vi "Frequency_Counter_TTi_SoftFP.vi"(0 "reference in":refnum<class "Frequency_Counter_TTi.lvclass">, 2 "Floating":bool, 5 "error in (no error)":errorcluster) -> (14 "reference out":refnum<class "Frequency_Counter_TTi.lvclass">, 19 "error out":errorcluster)   [LabVIEW 2022 SP3, in "Frequency_Counter_TTi.lvlib" / "Frequency_Counter_TTi.lvclass"]
uses:
  Frequency_Counter_TTi.lvclass
  <vilib>/numeric/Random Number (Range) DBL.vi
  Components/ViPER.lvlibp/ViPER.lvclass
  <vilib>/measure/NI_MABase.lvlib
  C:/Projects/Medulla/ViPER/Examples/Flux_Capacitor_Tester/Components/ViPER.lvlibp/ViPER.lvclass
panel:
  in  "Measure":bool
  out "Waveform Graph":waveform(dbl)(graph)
  out "Freq MHz":dbl format="%.4f"
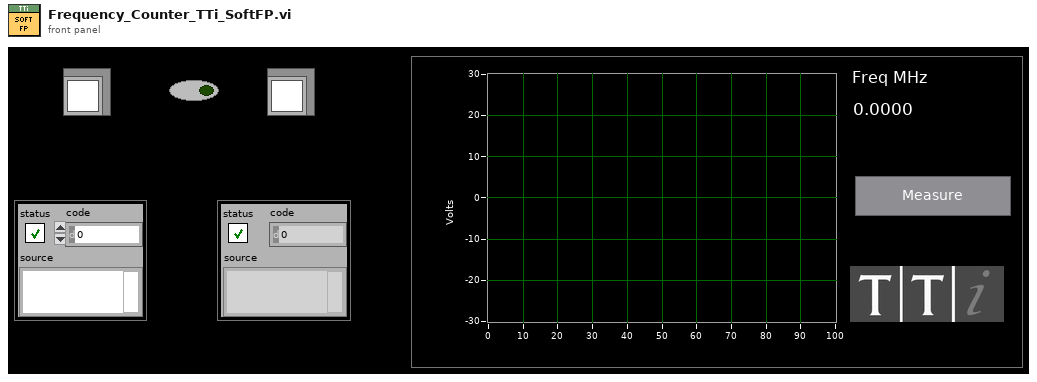
[diagram p1: front panel]
types:
  T1 = enum32{"Invalid", "Standard", "Closed", "Hidden", "Minimized", "Maximized"}
  T2 = enum16{"Sine Wave", "Triangle Wave", "Square Wave", "Sawtooth Wave"}[]
  T3 = typedef "Frequency_Counter_TTi.lvlib/Frequency_Counter_TTi.lvclass/ObjectAttributes.ctl" = cluster{"Config":T4, "Freq":dbl}
  T4 = typedef "Frequency_Counter_TTi.lvlib/Frequency_Counter_TTi.lvclass/Config.ctl" = cluster{"ComPort":refnum<visa-resource-name>}
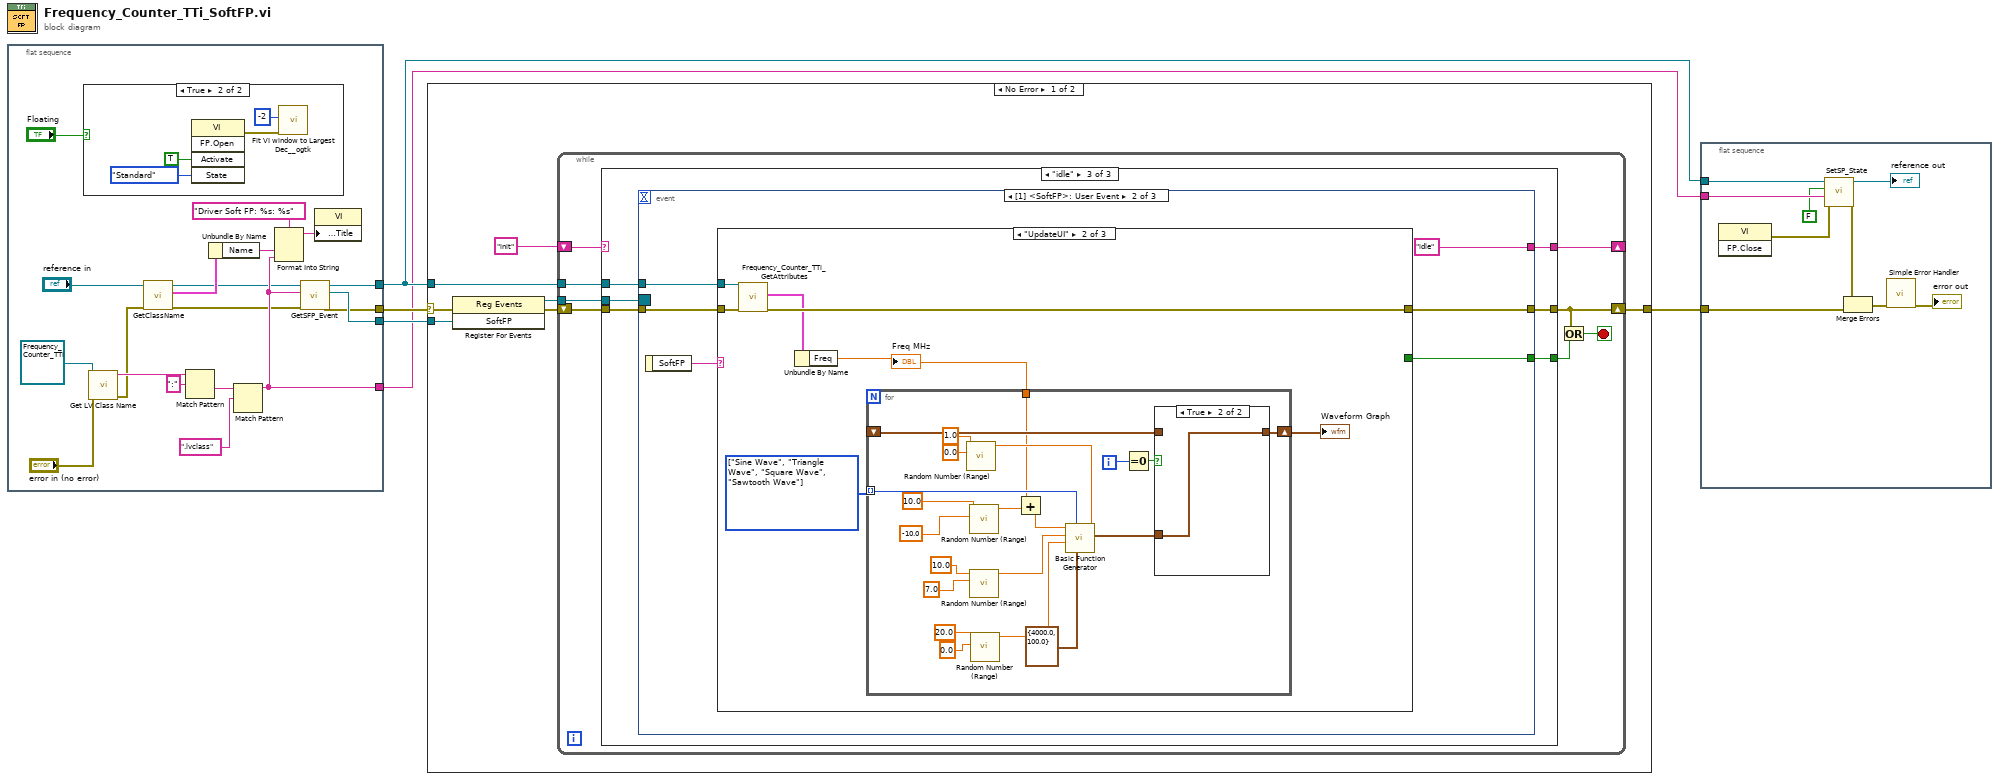
[diagram p0: block diagram]
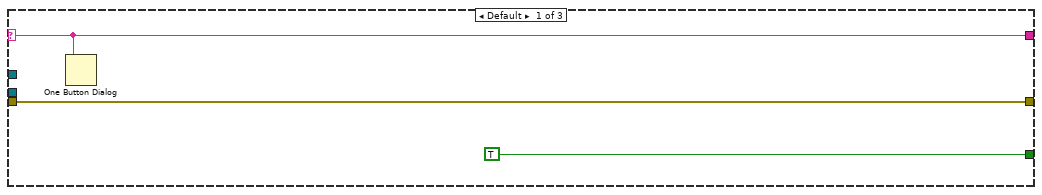
[diagram p3: hidden frame]
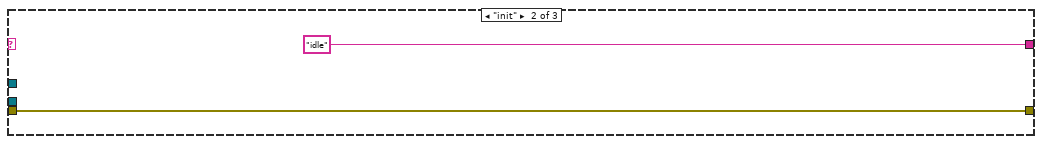
[diagram p4: hidden frame]
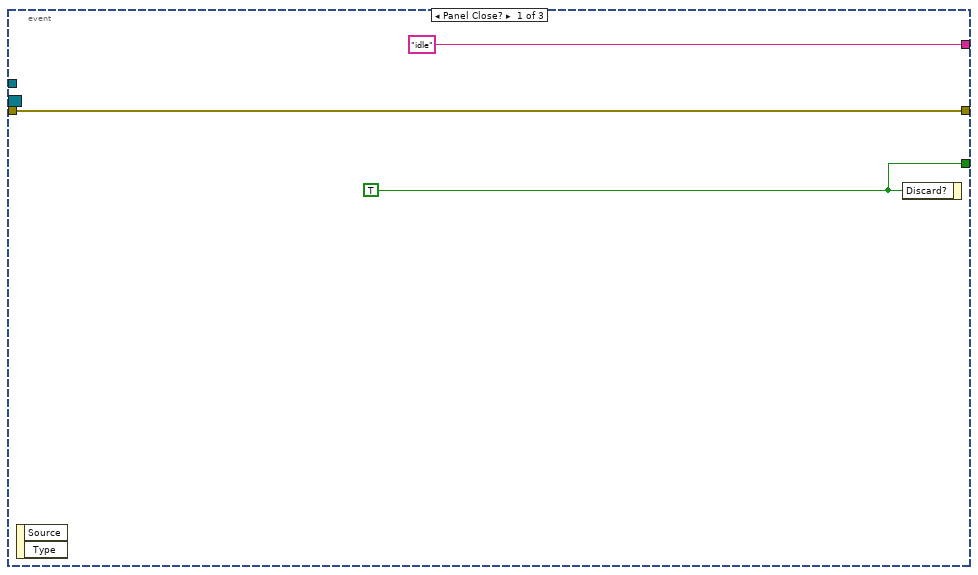
[diagram p5: hidden frame]
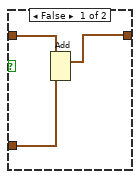
[diagram p7: hidden frame]
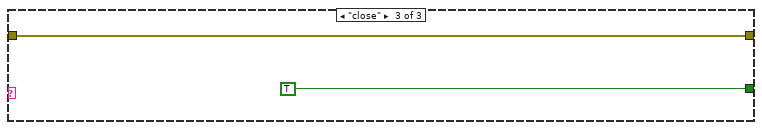
[diagram p8: hidden frame]
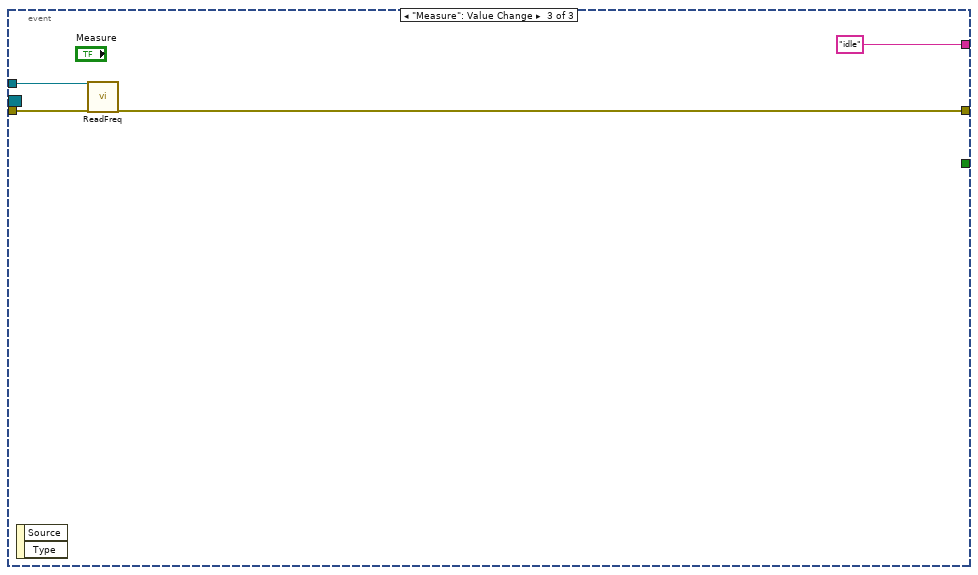
[diagram p9: hidden frame]
diagram:
  n1 = flat-sequence {
    tunnel: [w21] -> w5
    tunnel: [w20] -> w2
    tunnel: [w24] -> w3
    tunnel: [w12] -> w1
    frame #0 {
      n2 = case shown="True" "Floating" {
        frame False {
        }
        frame True {
          n3 = invoke class="VI" method="FP.Open"("Activate"=TRUE ("Activate?"), "State"=T1."Standard") -> (error out=w25:errorcluster)  [unwired: 3 in, 4 out]
          n4 = call <userlib>:"Fit VI window to Largest Dec__ogtk.vi"("error in (no error)"=w25, "border spacing (2 px)"=-2) -> ()  [unwired: 4 in, 2 out]
        }
      }
      n5 = call <vilib>:"Get LV Class Name.vi"("error in (no error)"="error in (no error)", "object"=refnum<class "Frequency_Counter_TTi.lvclass"> refnum ("reference")) -> ("error out"=w11:errorcluster, "class name"=w17:string)  [unwired: 8 in]
      n6 = call "GetClassName.vi"("error in (no error)"=w11, "reference in"="reference in") -> ("error out"=w10:errorcluster, "Details"=w9:cluster{"Name":string, "Class":string}, "reference out"=w7:refnum<class "Frequency_Counter_TTi.lvclass">)  [unwired: 7 in]
      n7 = Match Pattern(string=w17, regular expression=":") -> (after substring=w15:string)  [unwired: 1 in, 3 out]
      n8 = Unbundle By Name(w9) -> ("Name"=w19:string)
      n9 = Match Pattern(string=w15, regular expression=".lvclass") -> (before substring=w12:string)  [unwired: 1 in, 3 out]
      n10 = Format Into String(format string="Driver Soft FP: %s: %s", w19, w12) -> (resulting string=w23:string)  [unwired: 2 in, 1 out]
      n11 = call-dynamic "GetSFP_Event.vi"("error in (no error)"=w10, "Ancestor"=w12, "reference in"=w7) -> ("error out"=w21:errorcluster, "SoftFP"=w24:refnum<user-event>, "reference out"=w20:refnum<class "Frequency_Counter_TTi.lvclass">)  [unwired: 6 in]
      n12 = property class="VI"("Front Panel.Title"=w23) -> ()  [unwired: 2 in, 2 out]
    }
  }
  n13 = case shown="No Error" w5 {
    selector: w5 -> [w33 w103]
    tunnel: [w29 w103] -> w4
    tunnel: w2 -> [w30 _]
    tunnel: w3 -> [w35 _]
    frame No Error {
      n14 = register-events(error in=w33, w35) -> (reference out=w34:refnum<event-registration>, error out=w32:errorcluster)  [unwired: 1 in]
      n15 = while {
        shift-right: [w40] -> w29
        shift-left: w32 -> [w43]
        tunnel: w34 -> [w42]
        tunnel: w30 -> [w41]
        shift-right: [w36] -> _
        shift-left: "init" -> [w37]
        stop <- w39 stop-if-true
        n16 = case shown="\"idle\"" w37 {
          selector: w37 -> [w44 _ _]
          tunnel: w43 -> [w45 w47 w54]
          tunnel: w42 -> [_ _ w53]
          tunnel: w41 -> [_ _ w52]
          tunnel: [w45 w47 w51] -> w40
          tunnel: [TRUE ("Discard?") _ w50] -> w38
          tunnel: [w44 "idle" w49] -> w36
          frame Default {
            n17 = One Button Dialog(message=w44) -> ()  [unwired: 1 in, 1 out]
          }
          frame "init" {
          }
          frame "idle" {
            n18 = event shown="[1] <SoftFP>: User Event" {
              selector: w53 -> [_ _ _]
              dyn-events: _ -> [_ _ _]
              timeout: _ -> [_ _ _]
              tunnel: w54 -> [w57 w63 w100]
              tunnel: [w57 w61 w101] -> w51
              tunnel: [w56 w60 _] -> w50
              tunnel: w52 -> [_ w58 w99]
              tunnel: ["idle" "idle" "idle"] -> w49
              event Panel Close? {
                w56 = TRUE ("Discard?")
                n19 = event-data() -> ()  [unwired: 1 in, 2 out]
                n20 = event-data("Discard?"=w56) -> ()  [unwired: 1 in, 1 out]
              }
              event User Event {
                n21 = event-data() -> ("SoftFP"=w62:string)  [unwired: 1 in]
                n22 = case shown="\"UpdateUI\"" w62 {
                  tunnel: w63 -> [w64 w71 w98]
                  tunnel: [w64 w69 w98] -> w61
                  tunnel: [_ _ TRUE ("Discard?")] -> w60
                  tunnel: w58 -> [_ w70 _]
                  frame Default {
                  }
                  frame "UpdateUI" {
                    w66 = T2 [enum."Sine Wave", enum."Triangle Wave", enum."Square Wave", enum."Sawtooth Wave"] items=["Sine Wave", "Triangle Wave", "Square Wave", "Sawtooth Wave"]
                    n23 = call "Frequency_Counter_TTi_GetAttributes.vi"("error in (no error)"=w71, "reference in"=w70) -> ("error out"=w69:errorcluster, "Data"=w68:T3)  [unwired: 6 in, 2 out]
                    n24 = Unbundle By Name(w68) -> ("Freq"=w65:dbl)
                    "Freq MHz" <- w65
                    n25 = for {
                      tunnel: w66 -> [w80] mode=indexing
                      shift-right: [w78] -> w67
                      shift-left: _ -> [w77]
                      tunnel: w65 -> [w73]
                      i -> [w76]
                      n26 = call-poly <vilib>:"Random Number (Range).vi"("lower bound (0)"=0.0, "upper bound (100)"=1.0) -> ("number"=w81:dbl)  [unwired: 9 in]
                      n27 = call-poly <vilib>:"Random Number (Range).vi"("lower bound (0)"=-10.0 ("frequency"), "upper bound (100)"=10.0 ("frequency")) -> ("number"=w74:dbl)  [unwired: 9 in]
                      n28 = call-poly <vilib>:"Random Number (Range).vi"("lower bound (0)"=7.0, "upper bound (100)"=10.0) -> ("number"=w88:dbl)  [unwired: 9 in]
                      n29 = call-poly <vilib>:"Random Number (Range).vi"("lower bound (0)"=0.0 ("upper bound (100)"), "upper bound (100)"=20.0) -> ("number"=w85:dbl)  [unwired: 9 in]
                      n30 = Add(x=w73, y=w74) -> (x+y=w72:dbl)
                      n31 = call <vilib>:"Basic Function Generator.vi"("offset"=w81, "sampling info"=cluster{"Fs":dbl, "#s":dbl} {"Fs"=4000.0, "#s"=100.0}, "signal type"=w80, "phase"=w85, "amplitude"=w88, "frequency"=w72) -> ("signal out"=w79:waveform(dbl))  [unwired: 3 in, 2 out]
                      n32 = Equal To 0?(x=w76) -> (x = 0?=w75:bool)
                      n33 = case shown="True" w75 {
                        tunnel: w79 -> [w95 w96]
                        tunnel: [w94 w96] -> w78
                        tunnel: w77 -> [w93 _]
                        frame False {
                          n34 = Add(1:w95, 2:w93) -> (0:w94:waveform(dbl))  [unwired: 1 in, 1 out]
                        }
                        frame True {
                        }
                      }
                    }
                    "Waveform Graph" <- w67
                  }
                  frame "close" {
                  }
                }
              }
              event "Measure": Value Change {
                n35 = event-data() -> ()  [unwired: 1 in, 2 out]
                n36 = call-dynamic "ReadFreq.vi"("reference in"=w99, "error in (no error)"=w100) -> ("error out"=w101:errorcluster)  [unwired: 15 in, 2 out]
              }
            }
          }
        }
        n37 = Or(x=w40, y=w38) -> (x .or. y?=w39:bool)
      }
    }
    frame Error {
    }
  }
  n38 = flat-sequence {
    tunnel: w4 -> [w110]
    tunnel: w2 -> [w105]
    tunnel: w1 -> [w107]
    frame #0 {
      n39 = invoke class="VI" method="FP.Close"() -> (error out=w109:errorcluster)  [unwired: 3 in, 2 out]
      n40 = call "SetSP_State.vi"("error in (no error)"=w109, "Ancestor"=w107, "SP Open"=FALSE, "reference in"=w105) -> ("error out"=w108:errorcluster, "reference out"=→"reference out":refnum<class "Frequency_Counter_TTi.lvclass">)  [unwired: 6 in]
      n41 = Merge Errors(w108, w110) -> (w112:errorcluster)
      n42 = call <vilib>:"Simple Error Handler.vi"("error in (no error)"=w112) -> ("error out"=→"error out":errorcluster)  [unwired: 4 in, 4 out]
    }
  }
